vi "UE9 Multiple AIN Example.vi"() -> ()   [LabVIEW 2021]
panel:
  in  "Ranges":string[](array[string])=["LJ_rgBIP5V", "LJ_rgBIP5V"]
  in  "Channels":i32[](array[numeric])=[0, 1]
  out "Values Read":dbl[](array[numeric]) format="%.6f"
  out "Error Message":string
  in  "Resolution":i32=12
  out "error out":errorcluster
  # "Aquires multiple analog input channels over USB from the first found UE9."
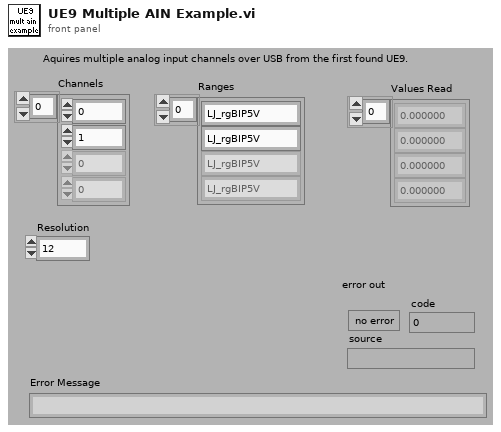
[diagram p1: front panel]
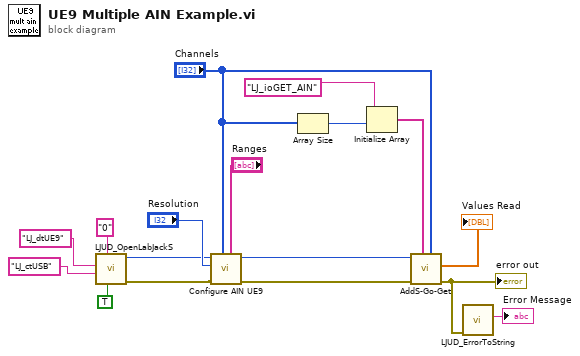
[diagram p0: block diagram]
diagram:
  n1 = call "LJUD_OpenLabJackS.vi"("FirstFound"=TRUE, "Address"="0", "ConnectionType"="LJ_ctUSB", "DeviceType"="LJ_dtUE9") -> ("error out"=w5:errorcluster, "Handle"=w6:i32)  [unwired: 5 in, 1 out]
  n2 = call "Configure AIN UE9.vi"("Ranges"="Ranges", "Channels"="Channels", "error in"=w5, "Resolution"="Resolution", "Handle In"=w6) -> ("error out"=w14:errorcluster, "Handle Out"=w15:i32)  [unwired: 5 in]
  n3 = Array Size(array="Channels") -> (size(s)=w2:i32)
  n4 = Initialize Array("LJ_ioGET_AIN" ("IOType"), w2) -> (w3:string[])
  n5 = call "AddS-Go-Get.vi"("Channels"="Channels", "IOTypes"=w3, "error in"=w14, "Handle In"=w15) -> ("error out"=w13:errorcluster, "Values Read"=→"Values Read":dbl[])  [unwired: 5 in, 1 out]
  "error out" <- w13
  n6 = call "LJUD_ErrorToString.vi"("error in"=w13) -> ("String"=→"Error Message":string)  [unwired: 10 in]
